vi "TIFF Error Handler.vi"(8 "error in (no error)":errorcluster, 11 "TIFF DLL error":i32) -> (0 "error out":errorcluster)   [LabVIEW 2012]
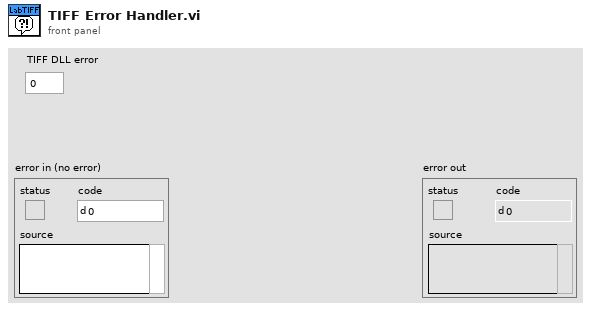
[diagram p1: front panel]
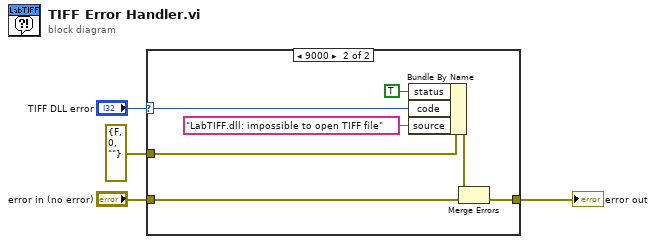
[diagram p0: block diagram]
diagram:
  n1 = case shown="9000" "TIFF DLL error" {
    selector: "TIFF DLL error" -> [_ w8]
    tunnel: [w5 w9] -> w3
    tunnel: "error in (no error)" -> [w5 w11]
    tunnel: errorcluster {"status"=FALSE, "code"=0, "source"=""} ("error constant") -> [_ w12]
    frame 0, Default {
    }
    frame 9000 {
      n2 = Bundle By Name(cluster=w12, "status"=TRUE, "code"=w8, "source"="LabTIFF.dll: impossible to open TIFF file") -> (w10:errorcluster)
      n3 = Merge Errors(w10, w11) -> (w9:errorcluster)
    }
  }
  "error out" <- w3
